vi "Main.vi"() -> ()   [LabVIEW 2014]
uses:
  Controls/Query.ctl
  <vilib>/DataFinder/DataTypes/object type.ctl
  <vilib>/DataFinder/DataTypes/comparison operator.ctl
  Controls/PolarSelectorRev.ctl
  Controls/ShowCoolingTrend.ctl
  Controls/ShowWarmingTrend.ctl
  <vilib>/userdefined/High Color/DFDataFinder.ctl
  Controls/DFQuery.ctl
  <vilib>/DataFinder/Close Reference (Query).vi
  <vilib>/DataFinder/Close Reference (DataFinder).vi
  <vilib>/Analysis/NI_AALPro.lvlib
  <vilib>/DataFinder/NI_DataFinder Toolkit.lvlib
  <vilib>/userdefined/NI_DataFinder Controls.lvlib
panel:
  out "error out":errorcluster
  in  "Show":bool
  in  "Stop Button":bool
  in  "Previous Button":bool
  in  "Next Button":bool
  in  "Needle Spacing":i16=85
  out "Submit Query":bool
  in  "Tab Control":enum32{"Acquire", "Analyze", "Visualize"}(tab)
  in  "File to Display":i32(listbox)
  out "Temperature, Pressure, Wind Speed, Wind Direction":dynamicdata(graph)
  in  "Queries":T1=[{"Object Type"=2, "Property Name"="Name", "Operator"=0, "Value"="Temperature", "Enable Query?"=TRUE, "Radio Buttons"=enum."Radio Selection 1"}, {"Object Type"=1, "Property Name"="Longitude", "Operator"=2, "Value"="-45", "Enable Query?"=TRUE, "Radio Buttons"=enum."Radio Selection 2"}, {"Object Type"=1, "Property Name"="Longitude", "Operator"=3, "Value"="0", "Enable Query?"=TRUE, "Radio Buttons"=enum."Radio Selection 2"}, {"Object Type"=1, "Property Name"="MeasurementMonth", "Operator"=0, "Value"="July", "Enable Query?"=TRUE, "Radio Buttons"=enum."Radio Selection 1"}] {"Object Type" items=["File", "Channel Group", "Channel"]; "Operator" items=["=", "<>", ">", "<", ">=", "<=", "#"]}
  out "Search Results":string[][](table) caption="Search Results (95)"
  in  "Search":bool
  out "Deg C/Year (Antarctica)":dbl
  in  "Warming Trend":T4
  in  "Cooling Trend":T5
  in  "Load Austin Data":bool
  in  "Dial":T6={-45, 0} scale=-180.0..180.0
  out "Antarctica":T7(graph)
  out "Deg C/Year (Austin)":dbl
  out "Austin":T8(graph)
  # "1. Acquire Data quickly"
  # "2. Analyze Data programmatically"
  # "3. Visualize Results insightfully"
  # "Drag the needles and scroll the mouse wheel to change the query."
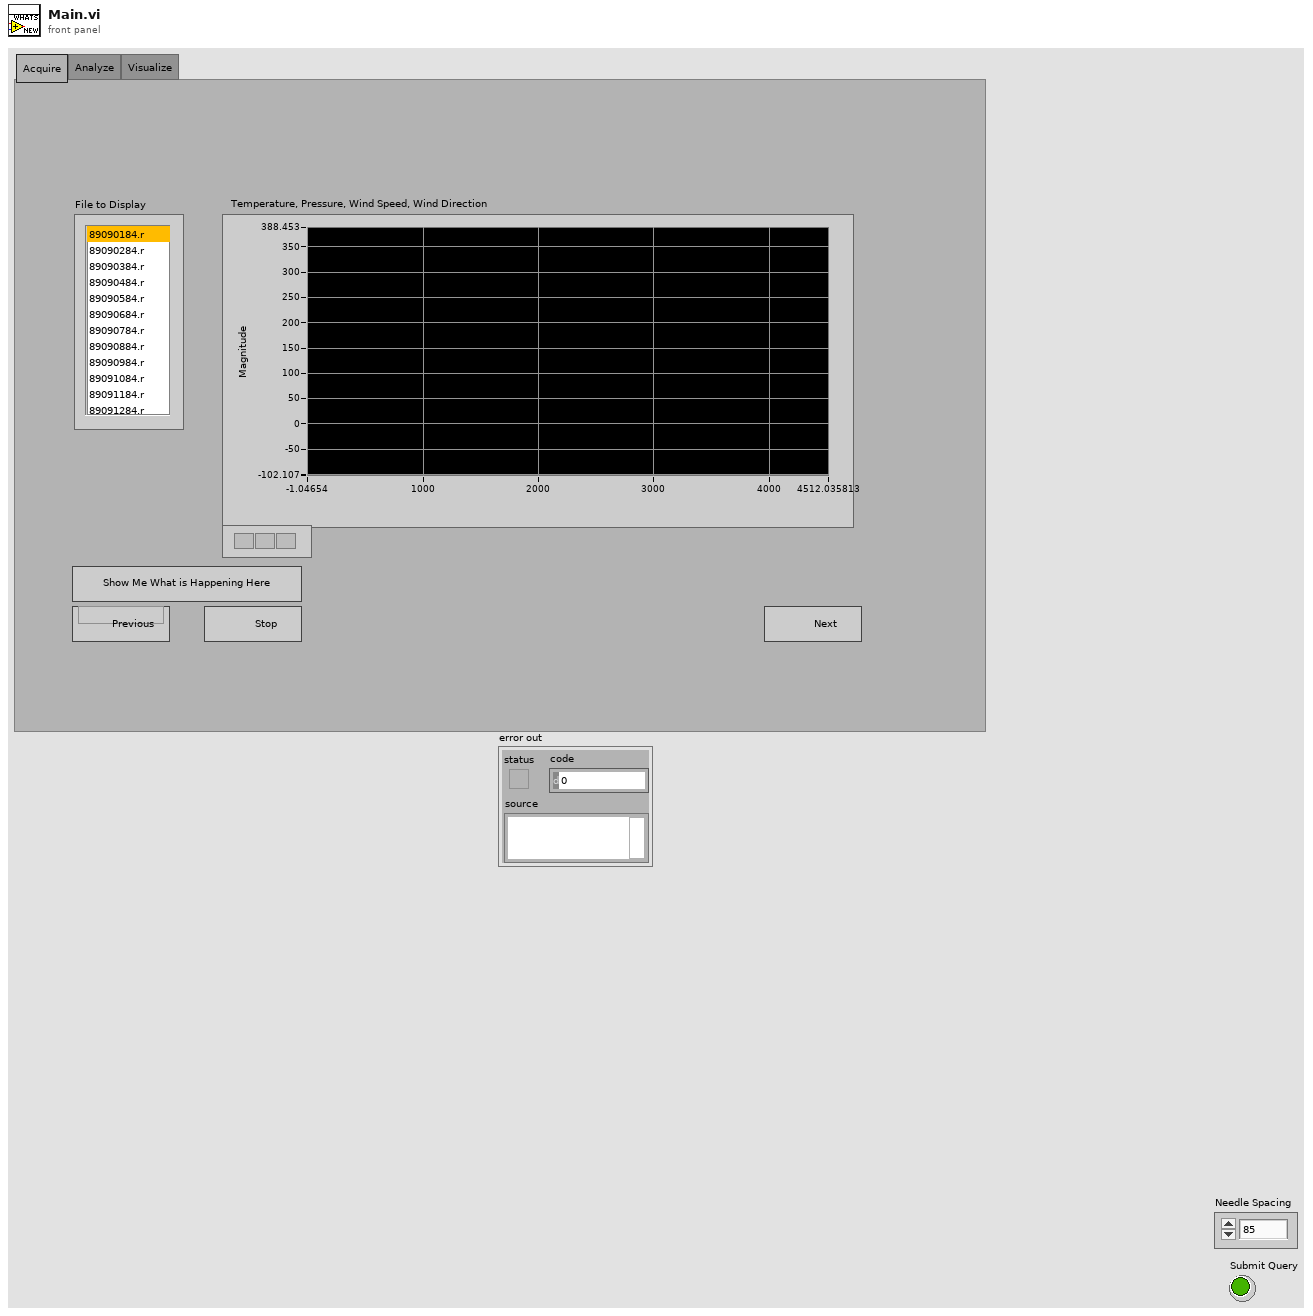
[diagram p1: front panel]
types:
  T1 = typedef "Query.ctl" = cluster{"Object Type":T2, "Property Name":string, "Operator":T3, "Value":string, "Enable Query?":bool, "Radio Buttons":enum32{"Radio Selection 1", "Radio Selection 2"}}[]
  T2 = typedef "NI_DataFinder Toolkit.lvlib/object type.ctl" = u16
  T3 = typedef "NI_DataFinder Toolkit.lvlib/comparison operator.ctl" = u16
  T4 = typedef "ShowWarmingTrend.ctl" = bool
  T5 = typedef "ShowCoolingTrend.ctl" = bool
  T6 = typedef "PolarSelectorRev.ctl" = cluster{i16, i16}
  T7 = cluster{"property values":timestamp[], "Best Linear Fit":dbl[]}[]
  T8 = cluster{"Year":i32[], "Average Temp Array":dbl[]}[]
  T9 = typedef "NI_DataFinder Controls.lvlib/DFDataFinder.ctl" = refnum<k21>
  T10 = typedef "DFQuery.ctl" = cluster{"Object Type":T2, "Property Name":string, "Operator":T3, "Value":string, "Enable Query?":bool, "Radio Buttons":enum32{"Radio Selection 1", "Radio Selection 2"}}[]
  T11 = typedef "NI_DataFinder Controls.lvlib/DFQuery.ctl" = refnum<k20>
  T12 = typedef "NI_DataFinder Controls.lvlib/DFSearchResult.ctl" = refnum<k20>
  T13 = typedef "NI_DataFinder Toolkit.lvlib/results elements.ctl" = cluster{"fullpaths":path[], "DataPlugin names":string[], "channel group names":string[], "channel names":string[]}
  T14 = cluster{"Object Type":T2, "Property Name":string, "Operator":T3, "Value":string, "Enable Query?":bool, "Radio Buttons":enum32{"Radio Selection 1", "Radio Selection 2"}}
  T15 = cluster{"Year":i32[], "Average Temp Array":dbl[]}
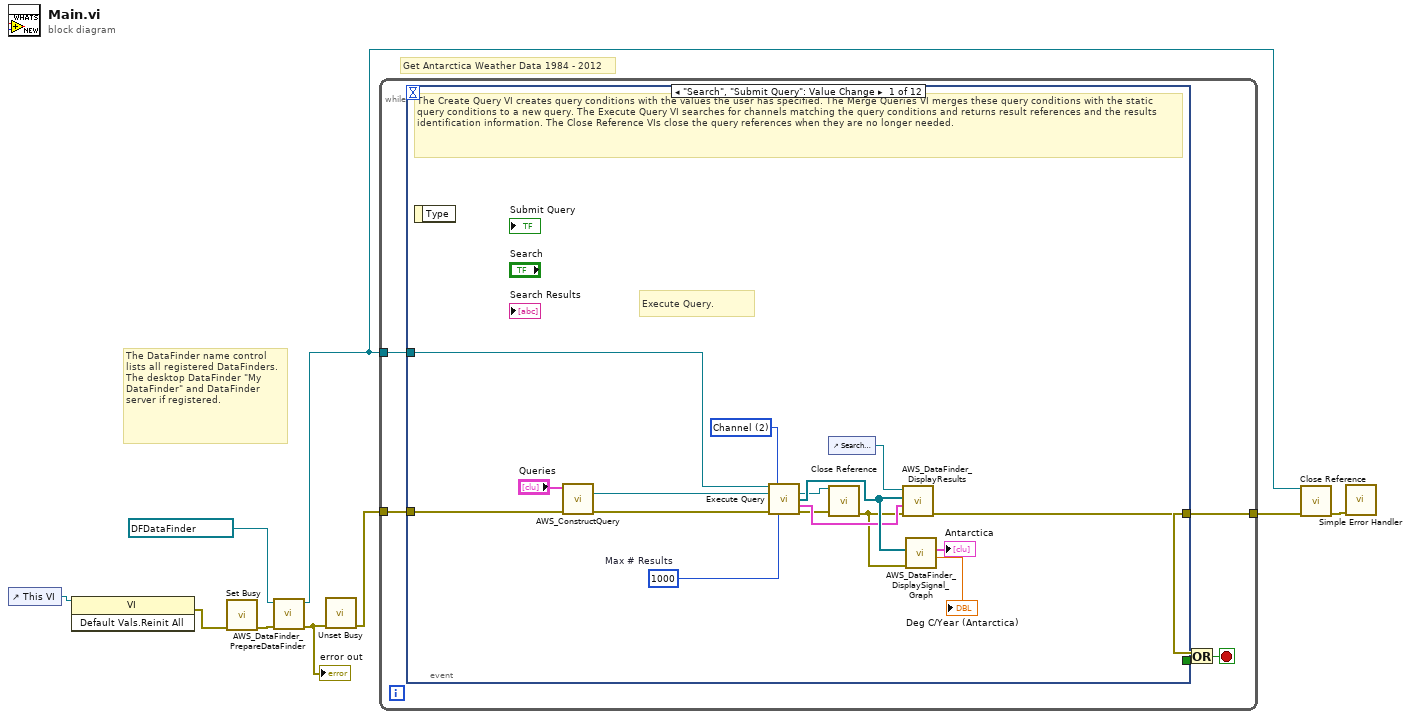
[diagram p0: block diagram]
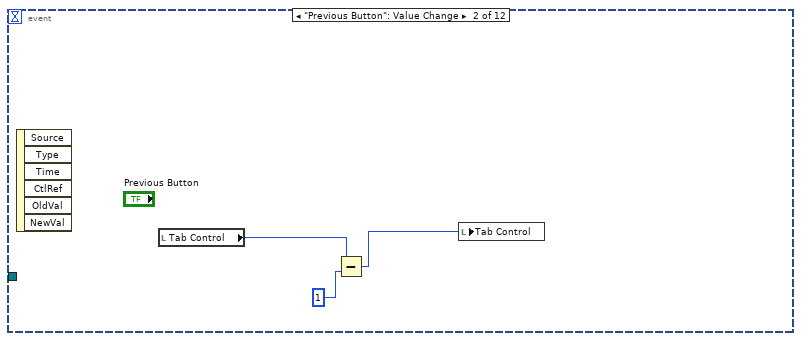
[diagram p2: hidden frame]
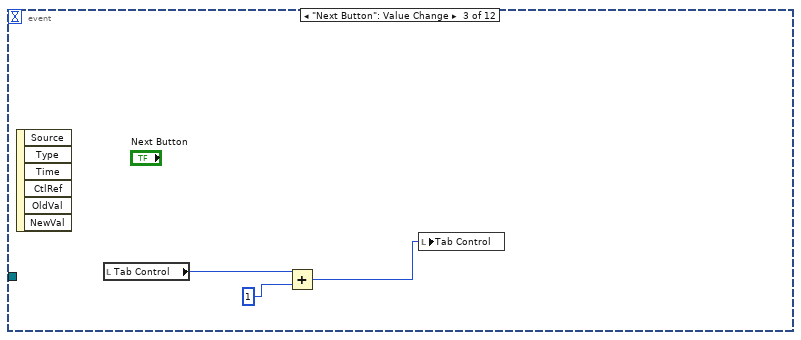
[diagram p3: hidden frame]
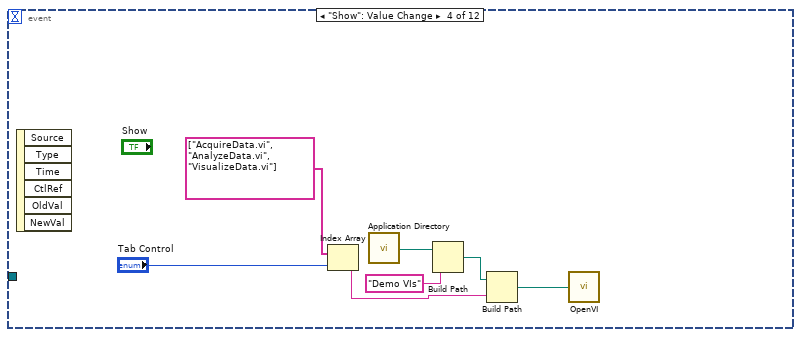
[diagram p4: hidden frame]
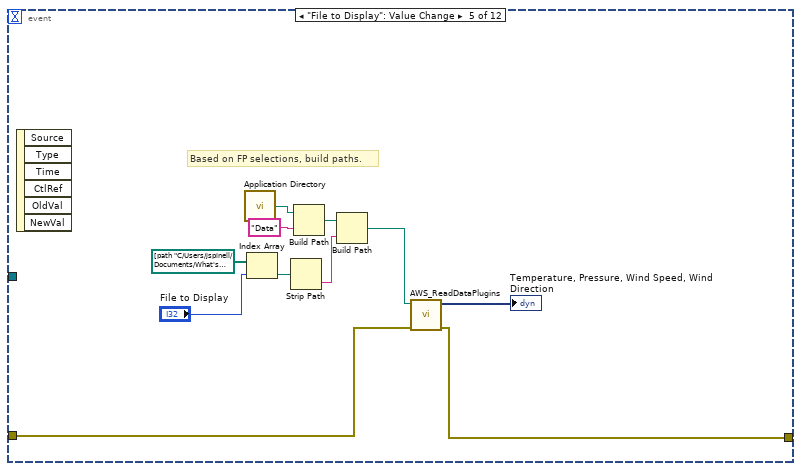
[diagram p5: hidden frame]
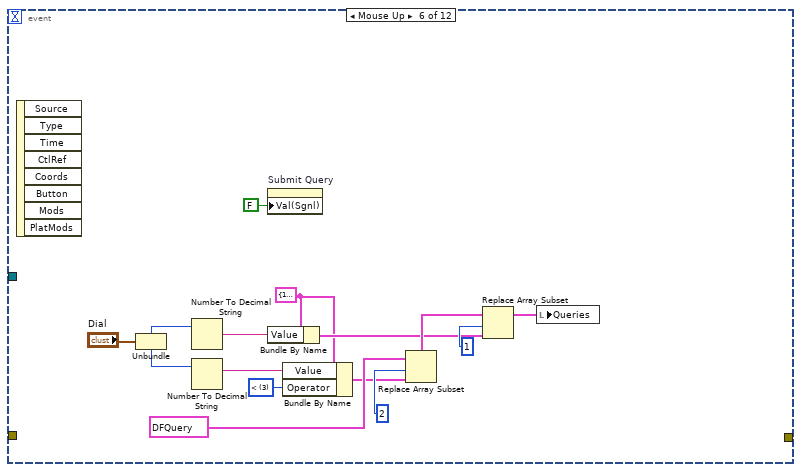
[diagram p6: hidden frame]
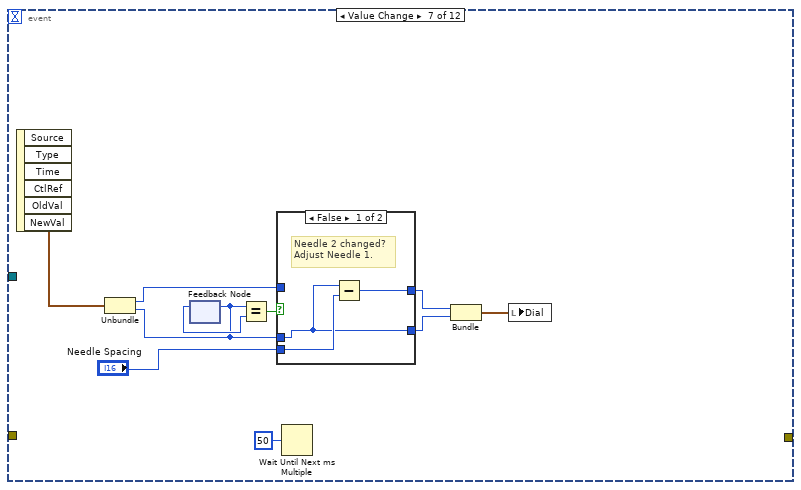
[diagram p7: hidden frame]
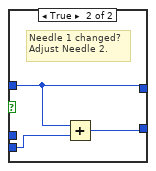
[diagram p8: hidden frame]
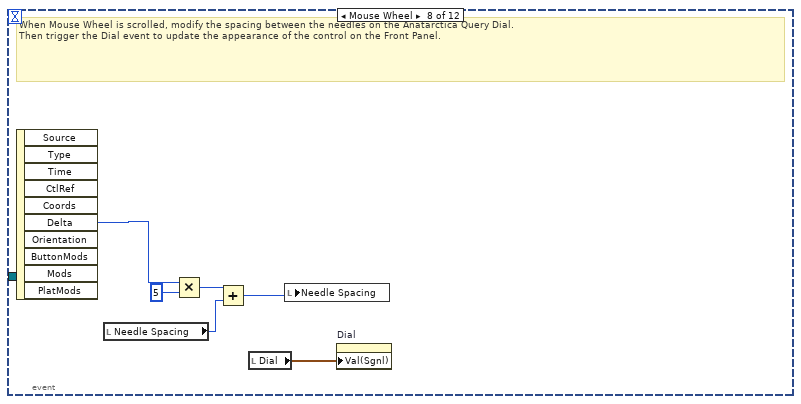
[diagram p9: hidden frame]
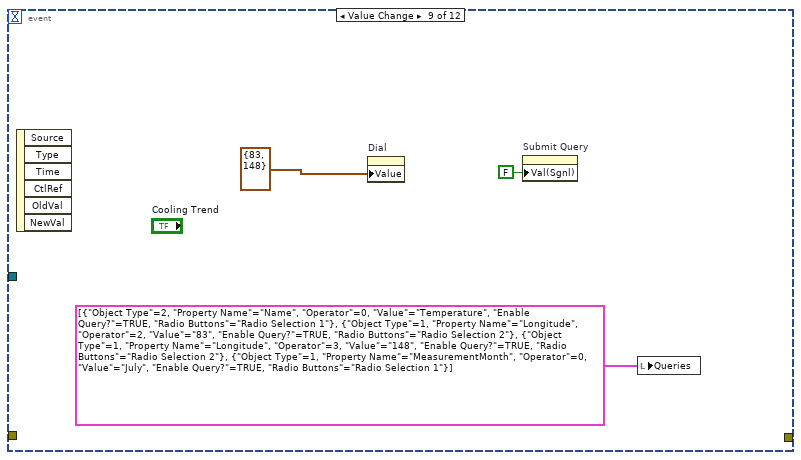
[diagram p10: hidden frame]
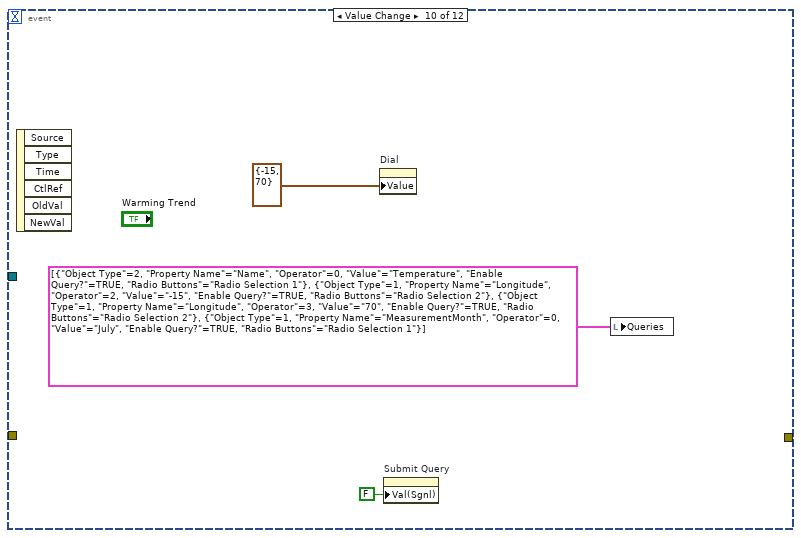
[diagram p11: hidden frame]
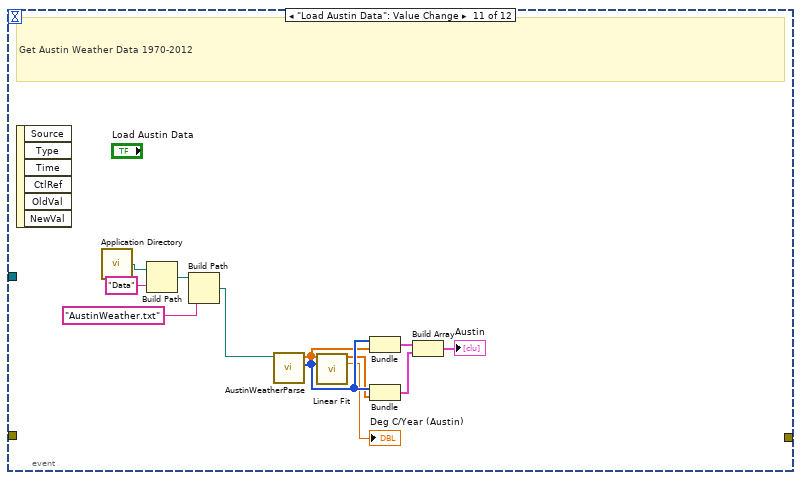
[diagram p12: hidden frame]
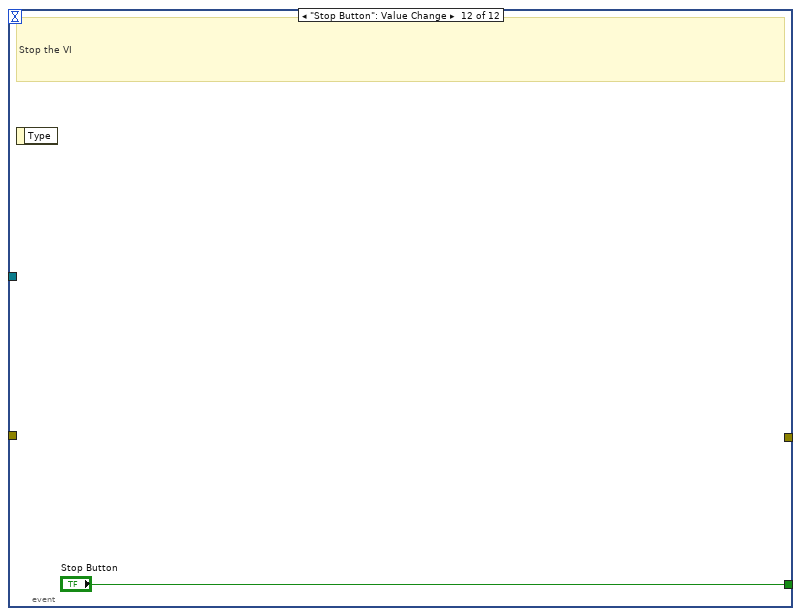
[diagram p13: hidden frame]
diagram:
  # "The DataFinder name control lists all registered DataFinders. The desktop DataFinder \"My DataFinder\" and DataFinder server if registered."
  # "Get Antarctica Weather Data 1984 - 2012"
  n1 = control-ref of="This VI"() -> (w3:refnum<vi>)
  n2 = invoke class="VI" method="Default Vals.Reinit All"(reference=w3) -> (error out=w2:errorcluster)  [unwired: 2 in, 2 out]
  n3 = call <vilib>:"Set Busy.vi"("error in (no error)"=w2) -> ("error out"=w6:errorcluster)  [unwired: 9 in, 1 out]
  n4 = call "AWS_DataFinder_PrepareDataFinder.vi"("error in"=w6, "DataFinder"=T9 "My DataFinder") -> ("error out"=w5:errorcluster, "DataFinder reference out"=w4:T9)  [unwired: 8 in]
  "error out" <- w5
  n5 = call <vilib>:"Unset Busy.vi"("error in (no error)"=w5) -> ("error out"=w7:errorcluster)  [unwired: 10 in]
  n6 = while {
    tunnel: w4 -> [w14]
    tunnel: [w11] -> w9
    tunnel: w7 -> [w10]
    stop <- w13 stop-if-true
    n7 = event shown="[0] \"Search\", \"Submit Query\": Value Change" {
      selector: _ -> [_ _ _ _ _ _ _ _ _ _ _ _]
      dyn-events: _ -> [_ _ _ _ _ _ _ _ _ _ _ _]
      timeout: _ -> [_ _ _ _ _ _ _ _ _ _ _ _]
      tunnel: [_ _ _ _ _ _ _ _ _ _ _ "Stop Button"] -> w12
      tunnel: w14 -> [w29 _ _ _ _ _ _ _ _ _ _ _]
      tunnel: [w30 _ _ _ w50 _ _ _ _ _ _ _] -> w11
      tunnel: w10 -> [w28 _ _ _ w51 _ _ _ _ _ _ _]
      event "Search", "Submit Query": Value Change {
        w19 = u32 1000  # Max # Results
        w22 = T2 2 items=["File", "Channel Group", "Channel"] ("Object Type 2")
        # "Execute Query."
        # "The Create Query VI creates query conditions with the values the user has specified. The Merge Queries VI merges these query conditions with the static query conditions to a new query. The Execute Query VI searches for channels matching the query conditions and returns result references and the results identification information. The Close Reference VIs close the query references when they are no longer needed."
        n8 = event-data() -> ()  [unwired: 2 out]
        n9 = call "AWS_ConstructQuery.vi"("error in (no error)"=w28, "Queries"="Queries") -> ("error out"=w20:errorcluster, "Refnum out"=w18:T11)  [unwired: 8 in]
        n10 = call <vilib>:"Execute Query.vi"("DataFinder reference"=w29, "result object type (file)"=w22, "query reference"=w18, "error in (no error)"=w20, "max results count (200)"=w19) -> ("query reference out"=w24:T11, "result references out"=w27:T12[], "results elements"=w26:T13, "error out"=w23:errorcluster)  [unwired: 1 in, 6 out]
        n11 = control-ref of="Search Results"() -> (w25:refnum<vi>)
        n12 = call-poly <vilib>:"Close Reference.vi"("query reference"=w24, "error in (no error)"=w23) -> ("error out"=w17:errorcluster)  [unwired: 13 in]
        n13 = call "AWS_DataFinder_DisplayResults.vi"("error in"=w17, "results elements"=w26, "result references"=w27, "Tbl Refnum"=w25) -> ("error out"=w30:errorcluster)  [unwired: 6 in, 1 out]
        n14 = call "AWS_DataFinder_DisplaySignal_Graph.vi"("error in"=w17, "result references"=w27) -> ("slope"=→"Deg C/Year (Antarctica)":dbl, "XY Graph"=→"Antarctica":T7)  [unwired: 7 in, 1 out]
      }
      event "Previous Button": Value Change {
        n15 = event-data() -> ()  [unwired: 7 out]
        n16 = local read "Tab Control"() -> (w33:enum32{"Acquire", "Analyze", "Visualize"})
        n17 = Subtract(x=w33, y=1) -> (x-y=w31:u32)
        n18 = local write "Tab Control"(w31) -> ()
      }
      event "Next Button": Value Change {
        n19 = event-data() -> ()  [unwired: 7 out]
        n20 = local read "Tab Control"() -> (w36:enum32{"Acquire", "Analyze", "Visualize"})
        n21 = Add(x=w36, y=1) -> (x+y=w34:u32)
        n22 = local write "Tab Control"(w34) -> ()
      }
      event "Show": Value Change {
        n23 = event-data() -> ()  [unwired: 7 out]
        n24 = Index Array(array=string[] ["AcquireData.vi", "AnalyzeData.vi", "VisualizeData.vi"], index="Tab Control") -> (element=w37:string)
        n25 = call <vilib>:"Application Directory.vi"() -> ("Application Directory"=w43:path)
        n26 = Build Path(base path=w43, name or relative path="Demo VIs") -> (appended path=w40:path)
        n27 = Build Path(base path=w40, name or relative path=w37) -> (appended path=w39:path)
        n28 = call "OpenVI.vi"("vi path"=w39) -> ()
      }
      event "File to Display": Value Change {
        # "Based on FP selections, build paths."
        n29 = event-data() -> ()  [unwired: 7 out]
        n30 = call <vilib>:"Application Directory.vi"() -> ("Application Directory"=w49:path)
        n31 = Index Array(array=path[] [path "C:/Users/jspinell/Documents/What's New Demo/1984/89090184.r", path "C:/Users/jspinell/Documents/What's New Demo/1984/89090284.r", path "C:/Users/jspinell/Documents/What's New Demo/1984/89090384.r", path "C:/Users/jspinell/Documents/What's New Demo/1984/89090484.r", path "C:/Users/jspinell/Documents/What's New Demo/1984/89090584.r", path "C:/Users/jspinell/Documents/What's New Demo/1984/89090684.r", path "C:/Users/jspinell/Documents/What's New Demo/1984/89090784.r", path "C:/Users/jspinell/Documents/What's New Demo/1984/89090884.r", path "C:/Users/jspinell/Documents/What's New Demo/1984/89090984.r", path "C:/Users/jspinell/Documents/What's New Demo/1984/89091084.r", path "C:/Users/jspinell/Documents/What's New Demo/1984/89091184.r", path "C:/Users/jspinell/Documents/What's New Demo/1984/89091284.r"] ("Array"), index="File to Display") -> (element=w47:path)
        n32 = Strip Path(path=w47) -> (name=w46:string)  [unwired: 1 out]
        n33 = Build Path(base path=w49, name or relative path="Data") -> (appended path=w45:path)
        n34 = Build Path(base path=w45, name or relative path=w46) -> (appended path=w44:path)
        n35 = call "AWS_ReadDataPlugins.vi"("Error In"=w51, "File Path Control"=w44) -> ("Error Out"=w50:errorcluster, "Data Graph"=→"Temperature, Pressure, Wind Speed, Wind Direction":dynamicdata)  [unwired: 8 in]
      }
      event Mouse Up {
        w58 = T3 3 items=["=", "<>", ">", "<", ">=", "<=", "#"] ("Operator")
        w63 = T14 {"Object Type"=1, "Property Name"="Longitude", "Operator"=2, "Value"="", "Enable Query?"=TRUE, "Radio Buttons"=enum."Radio Selection 2"} ("new element/subarray")
        n36 = event-data() -> ()  [unwired: 9 out]
        n37 = Unbundle("Dial") -> (w56:i16, w57:i16)
        n38 = Number To Decimal String(number=w56) -> (decimal integer string=w65:string)  [unwired: 1 in]
        n39 = Number To Decimal String(number=w57) -> (decimal integer string=w59:string)  [unwired: 1 in]
        n40 = property on="Submit Query" class="Bool (strict)"("Val(Sgnl)"=FALSE ("Value (Signaling)")) -> ()  [unwired: 2 in, 2 out]
        n41 = Bundle By Name(cluster=w63, "Value"=w65) -> (w64:T14)
        n42 = Bundle By Name(cluster=w63, "Value"=w59, "Operator"=w58) -> (w62:T14)
        n43 = Replace Array Subset(array=T10 [{"Object Type"=2, "Property Name"="Name", "Operator"=0, "Value"="Temperature", "Enable Query?"=TRUE, "Radio Buttons"=enum."Radio Selection 1"}, {"Object Type"=1, "Property Name"="Longitude", "Operator"=2, "Value"="-90", "Enable Query?"=TRUE, "Radio Buttons"=enum."Radio Selection 2"}, {"Object Type"=1, "Property Name"="Longitude", "Operator"=3, "Value"="0", "Enable Query?"=TRUE, "Radio Buttons"=enum."Radio Selection 2"}, {"Object Type"=1, "Property Name"="MeasurementMonth", "Operator"=0, "Value"="July", "Enable Query?"=TRUE, "Radio Buttons"=enum."Radio Selection 1"}] ("Queries"), new element=w62, index=2) -> (w66:T10)
        n44 = Replace Array Subset(array=w66, new element=w64, index=1) -> (w61:T10)
        n45 = local write "Queries"(w61) -> ()
      }
      event Value Change {
        n46 = event-data() -> ("NewVal"=w74:T6)  [unwired: 6 out]
        n47 = Unbundle(w74) -> (w78:i16, w75:i16)
        n48 = feedback #1() -> (w77:i16)  [unwired: 1 in]
        n49 = feedback-in #1(w75) -> ()
        n50 = Equal?(x=w75, y=w77) -> (x = y?=w76:bool)
        n51 = case shown="False" w76 {
          tunnel: w75 -> [w80 _]
          tunnel: [w80 w83] -> w72
          tunnel: w78 -> [_ w85]
          tunnel: [w81 w85] -> w73
          tunnel: "Needle Spacing" -> [w82 w84]
          frame False {
            # "Needle 2 changed?\nAdjust Needle 1."
            n52 = Subtract(x=w80, y=w82) -> (x-y=w81:i16)
          }
          frame True {
            # "Needle 1 changed?\nAdjust Needle 2."
            n53 = Add(x=w85, y=w84) -> (x+y=w83:i16)
          }
        }
        n54 = Wait Until Next ms Multiple(millisecond multiple=u32 50) -> ()  [unwired: 1 out]
        n55 = Bundle(w73, w72) -> (w71:cluster{i16, i16})  [unwired: 1 in]
        n56 = local write "Dial"(w71) -> ()
      }
      event Mouse Wheel {
        # "When Mouse Wheel is scrolled, modify the spacing between the needles on the Anatarctica Query Dial.\nThen trigger the Dial event to update the appearance of the control on the Front Panel."
        n57 = event-data() -> ("Delta"=w91:i32)  [unwired: 10 out]
        n58 = local read "Needle Spacing"() -> (w87:i16)
        n59 = Multiply(x=w91, y=5) -> (x*y=w89:i32)
        n60 = Add(x=w89, y=w87) -> (x+y=w88:i32)
        n61 = local read "Dial"() -> (w86:T6)
        n62 = local write "Needle Spacing"(w88) -> ()
        n63 = property on="Dial" class="Knob (strict)"("Val(Sgnl)"=w86) -> ()  [unwired: 2 in, 2 out]
      }
      event Value Change {
        n64 = event-data() -> ()  [unwired: 7 out]
        n65 = property on="Dial" class="Knob (strict)"("Value"=T6 {83, 148} ("Dial")) -> ()  [unwired: 2 in, 2 out]
        n66 = property on="Submit Query" class="Bool (strict)"("Val(Sgnl)"=FALSE ("Value (Signaling)")) -> ()  [unwired: 2 in, 2 out]
        n67 = local write "Queries"(T10 [{"Object Type"=2, "Property Name"="Name", "Operator"=0, "Value"="Temperature", "Enable Query?"=TRUE, "Radio Buttons"=enum."Radio Selection 1"}, {"Object Type"=1, "Property Name"="Longitude", "Operator"=2, "Value"="83", "Enable Query?"=TRUE, "Radio Buttons"=enum."Radio Selection 2"}, {"Object Type"=1, "Property Name"="Longitude", "Operator"=3, "Value"="148", "Enable Query?"=TRUE, "Radio Buttons"=enum."Radio Selection 2"}, {"Object Type"=1, "Property Name"="MeasurementMonth", "Operator"=0, "Value"="July", "Enable Query?"=TRUE, "Radio Buttons"=enum."Radio Selection 1"}] ("Queries")) -> ()
      }
      event Value Change {
        n68 = event-data() -> ()  [unwired: 7 out]
        n69 = property on="Dial" class="Knob (strict)"("Value"=T6 {-15, 70} ("Dial")) -> ()  [unwired: 2 in, 2 out]
        n70 = property on="Submit Query" class="Bool (strict)"("Val(Sgnl)"=FALSE ("Value (Signaling)")) -> ()  [unwired: 2 in, 2 out]
        n71 = local write "Queries"(T10 [{"Object Type"=2, "Property Name"="Name", "Operator"=0, "Value"="Temperature", "Enable Query?"=TRUE, "Radio Buttons"=enum."Radio Selection 1"}, {"Object Type"=1, "Property Name"="Longitude", "Operator"=2, "Value"="-15", "Enable Query?"=TRUE, "Radio Buttons"=enum."Radio Selection 2"}, {"Object Type"=1, "Property Name"="Longitude", "Operator"=3, "Value"="70", "Enable Query?"=TRUE, "Radio Buttons"=enum."Radio Selection 2"}, {"Object Type"=1, "Property Name"="MeasurementMonth", "Operator"=0, "Value"="July", "Enable Query?"=TRUE, "Radio Buttons"=enum."Radio Selection 1"}] ("Queries")) -> ()
      }
      event "Load Austin Data": Value Change {
        # "Get Austin Weather Data 1970-2012"
        n72 = event-data() -> ()  [unwired: 7 out]
        n73 = call <vilib>:"Application Directory.vi"() -> ("Application Directory"=w102:path)
        n74 = Build Path(base path=w102, name or relative path="Data") -> (appended path=w100:path)
        n75 = Build Path(base path=w100, name or relative path="AustinWeather.txt") -> (appended path=w98:path)
        n76 = call "AustinWeatherParse.vi"("file path (dialog if empty)"=w98) -> ("Year"=w106:i32[], "Average Temp Array"=w104:dbl[])  [unwired: 9 in]
        n77 = call <vilib>:"Linear Fit.vi"("Y"=w104, "X"=w106) -> ("Best Linear Fit"=w105:dbl[], "slope"=→"Deg C/Year (Austin)":dbl)  [unwired: 9 in, 3 out]
        n78 = Bundle("Year"=w106, "Average Temp Array"=w104) -> (w108:T15)  [unwired: 1 in]
        n79 = Bundle("Year"=w106, "Best Linear Fit"=w105) -> (w109:cluster{"Year":i32[], "Best Linear Fit":dbl[]})  [unwired: 1 in]
        n80 = Build Array(w108, w109) -> (→"Austin":cluster{"Year":i32[], "Best Linear Fit":dbl[]}[])
      }
      event "Stop Button": Value Change {
        # "Stop the VI"
        n81 = event-data() -> ()  [unwired: 2 out]
      }
    }
    n82 = Or(x=w11, y=w12) -> (x .or. y?=w13:bool)
  }
  n83 = call-poly <vilib>:"Close Reference.vi"("DataFinder reference"=w4, "error in (no error)"=w9) -> ("error out"=w8:errorcluster)  [unwired: 13 in]
  n84 = call <vilib>:"Simple Error Handler.vi"("error in (no error)"=w8) -> ()  [unwired: 4 in, 5 out]
